vi "Measurement.vi"(5 "error in":errorcluster) -> (19 "error out":errorcluster)   [LabVIEW 2011]
uses:
  GlobalSettings.vi
  Utilities/controls/ctlSeqFNs_PI_SysNr.ctl
panel:
  in  "valsZaxisMeasurement":T1
  in  "out":T2
  out "z vorgabe":i32
  out "z num scanner":i32
  out "y num scanner":i32
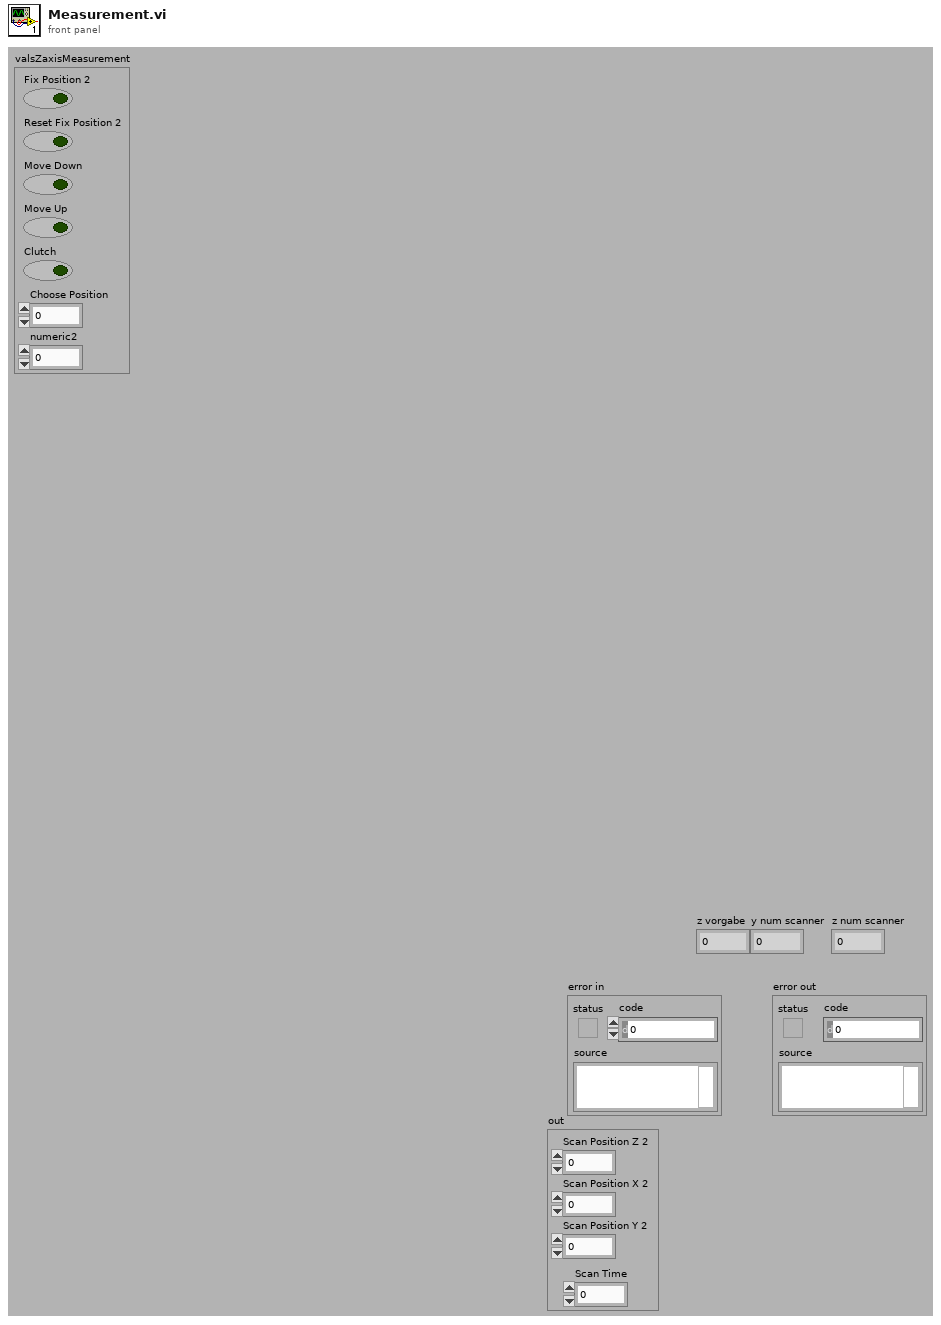
[diagram p1: front panel]
types:
  T1 = cluster{"Fix Position 2":bool, "Reset Fix Position 2":bool, "Move Down":bool, "Move Up":bool, "Clutch":bool, "Choose Position":dbl, "numeric2":dbl}
  T2 = cluster{"Scan Position Z 2":dbl, "Scan Position X 2":dbl, "Scan Position Y 2":dbl, "Scan Time":dbl}
  T3 = typedef "ctlSeqFNs_PI_SysNr.ctl" = enum16{"Zero", "E517", "E710"}
  T4 = cluster{"exposure":sgl, "accumulate":sgl, "kinetic":sgl}[]
  T5 = cluster{"exposure":sgl, "accumulate":sgl, "kinetic":sgl}
  T6 = cluster{"X-Min":dbl, "X-Len":dbl, "Y-Min":dbl, "Y-Len":dbl, "X-Delta":dbl, "Y-Delta ":dbl}
  T7 = cluster{"3d Layers_Num":dbl, "3d Start_Pos  Start":dbl, "3d Step_Delta_Layer":dbl}
  T8 = typedef "E517_Termination_character.ctl" = enum16{"LF", "CR", "LFCR", "CRLF"}
  T9 = typedef "E517_Controller_names.ctl" = enum16{"None", "Analog", "C-702", "C-843", "C-843.PM", "C-844", "C-848", "C-865", "C-866", "C-867", "C-880", "E-516", "E-517", "E-710", "E-712", "E-725", "E-753", "E-755", "E-761", "E-816", "E-861", "F-206", "M-840", "M-850", "M-8X0", "Mercury"}
  T10 = typedef "E517_Available_DLLs.ctl" = u16
  T11 = typedef "E517_Available_DLL_interfaces.ctl" = u16
  T12 = typedef "E517_Available_interfaces.ctl" = u16
  T13 = cluster{"Main-Global-Config out":cluster{"Global-Config":cluster{"DLL device ID's":i32[], "DLL Interface\nConfiguration":cluster{"DLL for Device":T10, "DLL Interface":T11, "Parameter":string}[], "Interface configuration":cluster{"RS232 Portnumber":i32, "Timeout":i32, "RS232 Baud rate":u32, "Interface":T12, "GPIB Bus":i32, "GPIB Address":i32, "GPIB Mode":i32}[], "Flow control":cluster{"input XON/XOFF":bool, "input HW Handshake":bool, "input alt HW HShk":bool, "output XON/XOFF":bool, "output HW Handshake":bool, "output alt HW HShk":bool, "XOFF byte ":u8, "XON byte":u8, "parity error byte":u16}[], "Bit settings and parity":cluster{"data bits":u16, "stop bits":enum16{"1 bit", "1.5 bits", "2 bits"}, "parity":enum16{"no parity", "odd parity", "even parity", "mark parity", "space parity"}}[], "TCP/IP Configuration":cluster{"Host address/name":string, "Port":i32, "Board":i32}[], "VISA Resource name":refnum<visa-resource-name>[], "Termination character":T8[], "Syntax":enum16{"GCS 1.0", "GCS 2.0"}[], "Logging mode":bool[], "Log file ref. no":refnum<file>[], "System no.":i32}, "DaisyChain configuration":cluster{"No. of devices":i32, "Port ID":i32, "Devices":string[], "Description":string}[], "System":cluster{"Conn. axes":string[], "Controller name":T9}[]}, "Axis-Status":cluster{"Online status (Array)?":bool[], "WG running?":bool[], "Servo status?":bool[]}, "Identification":string, "Conn. Axes":string[], "Position":dbl[], "+/- movement range":dbl[]}
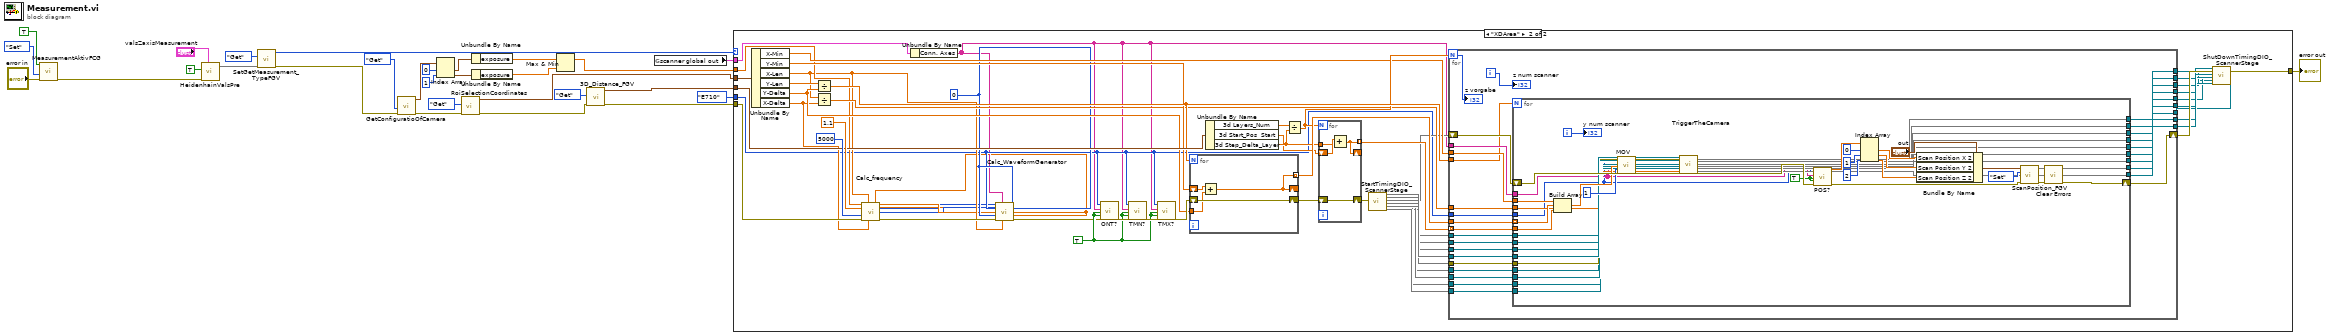
[diagram p0: block diagram]
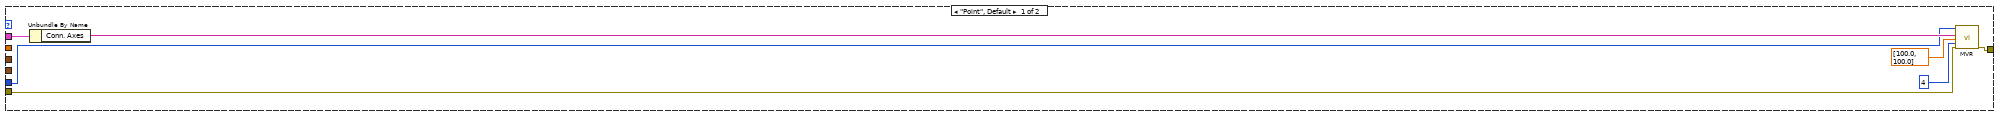
[diagram p2: hidden frame]
diagram:
  n1 = call "MeasurementAktivFCG.vi"("error in"="error in", "Set_Get"=enum16{"Set", "Get"}."Set", "Value"=TRUE) -> ("error out"=w5:errorcluster)  [unwired: 7 in, 1 out]
  n2 = call "HeidenhainValsPre.vi"(1:"valsZaxisMeasurement", 2:TRUE ("Reset Fix Position"), 5:w5) -> (6:w2)  [unwired: 5 in]
  n3 = call "SetGetMeasurement_TypeFGV.vi"("error in"=w2, "FGV_Control"=enum16{"Set", "Get"}."Get") -> ("error out"=w18:errorcluster, "Measurement Type 2"=w27:enum16{"Point", "XDArea"})  [unwired: 8 in]
  n4 = call "GetConfiguratioOfCamera.vi"("error in"=w18, "Set_Get"=enum16{"Set", "Get"}."Get") -> ("error out"=w17:errorcluster, "out"=w15:T4)  [unwired: 8 in]
  n5 = Index Array(array=w15, index #1=0 ("index"), index #2=1 ("index")) -> (element #1=w12:T5, element #2=w11:T5)
  n6 = call "RoiSelectionCoordinates.vi"("error in"=w17, "FGV_Control"=enum16{"Set", "Get"}."Get") -> ("error out"=w19:errorcluster, "ROI Coordinates out"=w24:T6)  [unwired: 8 in]
  n7 = Unbundle By Name(w12) -> ("exposure"=w10:sgl)
  n8 = Unbundle By Name(w11) -> ("exposure"=w9:sgl)
  n9 = Max & Min(x=w10, y=w9) -> (max(x,y)=w8:sgl)  [unwired: 1 out]
  n10 = call "3D_Distance_FGV.vi"("error in"=w19, "FGV_Control"=enum16{"Set", "Get"}."Get") -> ("error out"=w22:errorcluster, "3D out"=w20:T7)  [unwired: 8 in]
  n11 = global read "GlobalSettings.vi" "scanner global out"() -> (w28:T13)
  n12 = case shown="\"XDArea\"" w27 {
    tunnel: w22 -> [w36 w81]
    tunnel: w24 -> [_ w94]
    tunnel: [w30 w62] -> w25
    tunnel: w28 -> [w35 w89]
    tunnel: ctlSeqFNs_PI_SysNr."E710" ("DeviceNr.") -> [w33 w42]
    tunnel: w20 -> [_ w85]
    tunnel: w8 -> [_ w49]
    frame "Point", Default {
      n13 = Unbundle By Name(w35) -> ("Conn. Axes"=w34:string[])
      n14 = call "MVR.vi"("System no."=w33, "Axes to move"=w34, "Position values"=dbl[] [100.0, 100.0], "No.of digits"=i16 4, "error in"=w36) -> ("error out"=w30:errorcluster)  [unwired: 14 in]
    }
    frame "XDArea" {
      w44 = 0 ("X0")
      w83 = TRUE ("All axes?")
      n15 = Unbundle By Name(w94) -> ("X-Min"=w51:dbl, "Y-Min"=w75:dbl, "X-Len"=w45:dbl, "Y-Len"=w80:dbl, "Y-Delta"=w78:dbl, "X-Delta"=w52:dbl)
      n16 = Divide(x=w80, y=w78) -> (x/y=w79:dbl)
      n17 = Divide(x=w45, y=w52) -> (x/y=w50:dbl)
      n18 = call "Calc_frequency.vi"("ExitationTime In"=w49, "X-length"=w45, "CamTolerance"=1.1, "frequency in"=5000, "error in"=w81, "X-Delta"=w52) -> ("Wavepoints"=w38:dbl, "N"=w37:dbl, "TriggerLineCamWavepoints"=w43:dbl[], "divisor out"=w41:i32, "Array"=w40:u8[], "error out"=w47:errorcluster)  [unwired: 4 in]
      n19 = Unbundle By Name(w89) -> ("Conn. Axes"=w39:string[])
      n20 = call "Calc_WaveformGenerator.vi"("Scan parameters"=w41, "Wavepoint"=w39, "Trigger value 2"=w38, 3:w40, "wave table rate/ms"=w44, "System no."=w42, "scan time for 1 line/ms"=w44, 7:w43, 8:w37, 9:w44, 10:w37, "error in 2"=w47, 12:w45) -> ("error out 2"=w46:errorcluster)  [unwired: 2 in]
      n21 = call "ONT?.vi"("System no."=w42, "Axes to query"=w39, "All axes?"=w83, "Axis identifier?"=w83, "error in"=w46) -> ("error out"=w90:errorcluster)  [unwired: 13 in, 1 out]
      n22 = call "TMN?.vi"("System no."=w42, "Axes to query"=w39, "All axes?"=w83, "Axis identifier?"=w83, "error in"=w90) -> ("error out"=w91:errorcluster)  [unwired: 13 in, 1 out]
      n23 = call "TMX?.vi"("System no."=w42, "Axes to query"=w39, "All axes?"=w83, "Axis identifier?"=w83, "error in"=w91) -> ("error out"=w84:errorcluster)  [unwired: 13 in, 1 out]
      n24 = for {
        N: w79 -> [_]
        shift-right: [w174] -> _
        shift-left: w75 -> [w175]
        tunnel: [w174] -> w88 mode=indexing
        shift-right: [w173] -> w86
        shift-left: w84 -> [w173]
        tunnel: w78 -> [w172]
        n25 = Add(x=w175, y=w172) -> (x+y=w174:dbl)
      }
      n26 = Unbundle By Name(w85) -> ("3d Layers_Num"=w82:dbl, "3d Start_Pos  Start"=w74:dbl, "3d Step_Delta_Layer"=w77:dbl)
      n27 = Divide(x=w82, y=w77) -> (x/y=w76:dbl)
      n28 = for {
        N: w76 -> [_]
        shift-right: [w170] -> _
        shift-left: w74 -> [w171]
        tunnel: [w170] -> w87 mode=indexing
        shift-right: [w169] -> w73
        shift-left: w86 -> [w169]
        tunnel: w77 -> [w168]
        n29 = Add(x=w171, y=w168) -> (x+y=w170:dbl)
      }
      n30 = call "StartTimingDIO_ScannerStage.vi"(2:w73) -> (5:w70, 7:w69, 11:w71, 13:w64, 14:w67, 15:w65, 16:w48, 17:w66, 18:w72, 19:w68)  [unwired: 9 in]
      n31 = for {
        N: w76 -> [w117]
        tunnel: w39 -> [w123]
        tunnel: w42 -> [w122]
        tunnel: w88 -> [w121]
        tunnel: w51 -> [w120]
        tunnel: w87 -> [w119] mode=indexing
        shift-right: [w115] -> w63
        shift-left: w48 -> [w116]
        tunnel: w79 -> [w114]
        tunnel: w72 -> [w113]
        tunnel: w71 -> [w112]
        tunnel: w70 -> [w111]
        tunnel: w69 -> [w110]
        tunnel: w68 -> [w109]
        tunnel: w67 -> [w108]
        tunnel: w66 -> [w107]
        tunnel: w65 -> [w106]
        tunnel: w64 -> [w105]
        tunnel: [w104] -> w61
        tunnel: [w103] -> w60
        tunnel: [w102] -> w59
        tunnel: [w101] -> w58
        tunnel: [w100] -> w57
        tunnel: [w99] -> w56
        tunnel: [w98] -> w55
        tunnel: [w97] -> w54
        tunnel: [w96] -> w53
        tunnel: w50 -> [w95]
        i -> [w118]
        n32 = for {
          N: w114 -> [_]
          shift-right: [w167] -> w115
          shift-left: w116 -> [w166]
          tunnel: w122 -> [w125]
          tunnel: w123 -> [w126]
          tunnel: w121 -> [w163] mode=indexing
          tunnel: w120 -> [w162]
          tunnel: w119 -> [w161]
          tunnel: w113 -> [w145]
          tunnel: w112 -> [w144]
          tunnel: w111 -> [w143]
          tunnel: w110 -> [w142]
          tunnel: w109 -> [w141]
          tunnel: w108 -> [w140]
          tunnel: w107 -> [w139]
          tunnel: w106 -> [w138]
          tunnel: w105 -> [w137]
          tunnel: [w136] -> w104
          tunnel: [w135] -> w103
          tunnel: [w134] -> w102
          tunnel: [w133] -> w101
          tunnel: [w132] -> w100
          tunnel: [w131] -> w99
          tunnel: [w130] -> w98
          tunnel: [w129] -> w97
          tunnel: [w128] -> w96
          tunnel: w95 -> [w127]
          i -> [w160]
          w158 = TRUE ("Axis identifier?")
          n33 = Build Array(w162, w163, w161) -> (w164:dbl[])
          n34 = call "MOV.vi"("System no."=w125, "Axes to move"=w126, "Position values"=w164, "No.of digits"=i16 1, "error in"=w166) -> ("error out"=w124:errorcluster)  [unwired: 14 in]
          n35 = call "TriggerTheCamera.vi"(0:w145, 1:w141, 2:w140, 3:w139, 4:w138, 5:w137, 6:w127, "error out 2"=w124, 8:w144, 10:w143, 12:w142) -> (14:w128, 16:w129, 18:w130, 21:w131, 22:w132, 23:w133, 24:w134, 25:w135, 26:w136, "error out"=w159:errorcluster)  [unwired: 7 in]
          n36 = call "POS?.vi"("System no."=w125, "Axes to query"=w126, "All axes?"=w158, "Axis identifier?"=w158, "error in"=w159) -> ("Position"=w153:dbl[], "error out"=w157:errorcluster)  [unwired: 13 in]
          n37 = Index Array(array=w153, index #1=0 ("index"), index #2=1 ("index"), index #3=2 ("index")) -> (element #1=w151:dbl, element #2=w149:dbl, element #3=w147:dbl)
          n38 = Bundle By Name(cluster="out", "Scan Position X 2"=w151, "Scan Position Y 2"=w149, "Scan Position Z 2"=w147) -> (w154:T2)
          n39 = call "ScanPosition_FGV.vi"("error in"=w157, "FGV_Control"=enum16{"Set", "Get"}."Set", "in"=w154) -> ("error out"=w156:errorcluster)  [unwired: 7 in, 1 out]
          n40 = call <vilib>:"Clear Errors.vi"("error in (no error)"=w156) -> ("error out"=w167:errorcluster)  [unwired: 6 in]
          "y num scanner" <- w160
        }
        "z num scanner" <- w118
        "z vorgabe" <- w117
      }
      n41 = call "ShutDownTimingDIO_ScannerStage.vi"("task out 7"=w56, "error IO"=w63, "task out 2"=w61, "task out 3"=w60, "task out 5"=w58, "task out 9"=w55, "task out"=w53, "task out 10"=w54, "task out 6"=w57, "task out 4"=w59) -> ("error out"=w62:errorcluster)  [unwired: 9 in]
    }
  }
  "error out" <- w25
